vi "Test Coffee Shop Cashier Registers With Waiting to Order When Added.vi"(8 "error in (no error)":errorcluster, 11 "Coffee Shop Test in":refnum<class "Coffee Shop Test.lvclass">) -> (0 "error out":errorcluster, 3 "Coffee Shop Test out":refnum<class "Coffee Shop Test.lvclass">)   [LabVIEW 2020, in "Coffee Shop Test.lvclass"]
uses:
  Coffee Shop Test.lvclass
  C:/Program Files (x86)/National Instruments/LabVIEW 2020/vi.lib/Astemes/LUnit/Test Case.lvclass
  Processes/Coffee Shop/Coffee Shop.lvclass
  C:/Program Files (x86)/National Instruments/LabVIEW 2020/vi.lib/Astemes/Triarc Framework/Process/Process.lvclass
  Test Doubles/Mock Job Handler/Mock Job Handler.lvclass
  C:/Git/astemes-triarc-examples/Coffee Shop/Processes/People/Process Job/Job Handler.lvclass
  Processes/People/Person/Person.lvclass
  <vilib>/Astemes/Triarc Framework/Process/Process.lvclass/Process.ctl
  <vilib>/Astemes/LUnit/Test Case.lvclass/Test Case.ctl
  5b6f61c0-8826-472e-96ca-d4b217d1aee1.vi
  <vilib>/Astemes/Triarc Framework/Process/Private/SubVIs/Wait for finish.vi
  <vilib>/Astemes/Triarc Framework/Process/Private/SubVIs/Set Lifecycle State.vi
  <vilib>/Astemes/Triarc Framework/Process/Protected/Messaging/Send Message.vi
  <vilib>/Astemes/Triarc Framework/Process/Public/Lifecycle/Get Lifecycle State.vi
  <vilib>/Astemes/LUnit/Palette/Pass.vi
  <vilib>/Astemes/LUnit/Palette/Fail.vi
  <vilib>/Astemes/LUnit/Compare Variants.vi
  <vilib>/Astemes/LUnit/Describe Comparison.vi
  <vilib>/Astemes/LUnit/Set Assertion Type.vi
  <vilib>/Astemes/Triarc Framework/Process/Private/SubVIs/Handle Debug Data.vi
  <vilib>/Utility/error.llb/Clear Errors.vi
  <vilib>/Astemes/LUnit/Add test result.vi
  <vilib>/Astemes/LUnit/Variant to string.vi
  <vilib>/Astemes/Triarc Framework/Logging/Log Debug.vi
  <vilib>/AdvancedString/1D String Array to Delimited String.vi
  <vilib>/Utility/High Resolution Relative Seconds.vi
  <vilib>/Astemes/LUnit/LUnit Record Assertion Result.vi
  <vilib>/Astemes/LUnit/LUnit Aggregate Assertion Results.vi
  <vilib>/Astemes/LUnit/Method Result/LUnit Merge Status.vi
  <vilib>/Astemes/LUnit/LUnit Concatenate result strings.vi
  <vilib>/Utility/error.llb/Error Cluster From Error Code.vi
  <vilib>/Utility/Data Type/Get Type Information.vi
  <vilib>/Utility/LVClass/Get LV Class Name.vi
  <vilib>/Astemes/Triarc Framework/Process/Process.lvclass
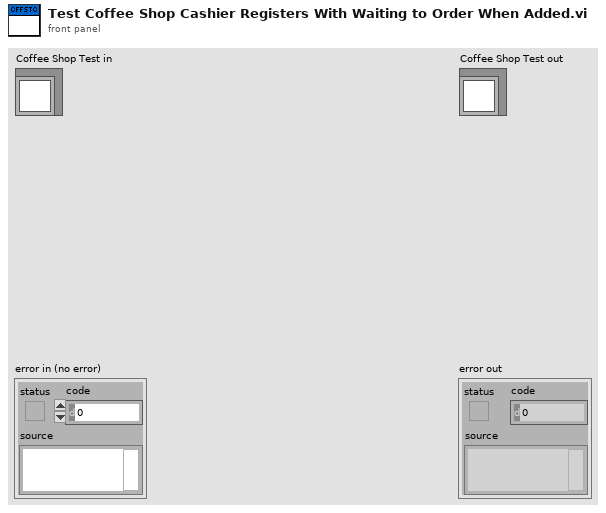
[diagram p1: front panel]
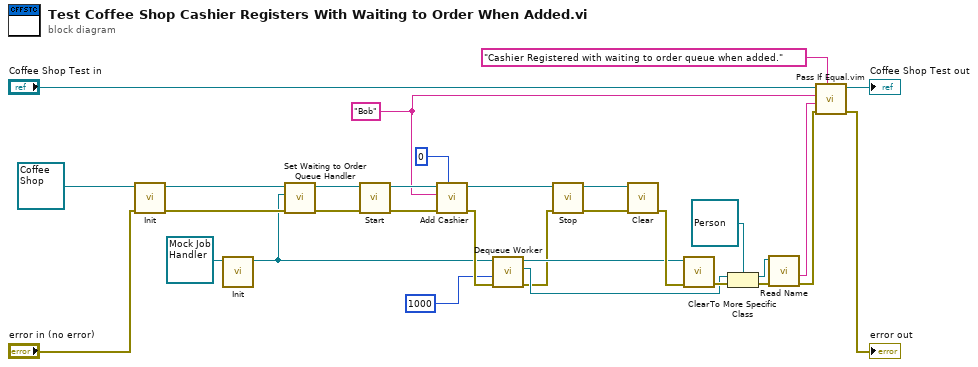
[diagram p0: block diagram]
diagram:
  w3 = "Bob" ("Name")
  n1 = call-dynamic "Init.vi"("error in (no error)"="error in (no error)", "Process In"=refnum<class "Coffee Shop.lvclass"> refnum ("Coffee Shop.lvclass")) -> ("error out"=w30:errorcluster, "Process Out"=w23:refnum<class "Coffee Shop.lvclass">)  [unwired: 8 in]
  n2 = call-dynamic "Init.vi"("Mock Job Handler In"=refnum<class "Mock Job Handler.lvclass"> refnum) -> ("Mock Job Handler Out"=w16:refnum<class "Mock Job Handler.lvclass">)  [unwired: 9 in, 1 out]
  n3 = call "Set Waiting to Order Queue Handler.vi"("error in (no error)"=w30, "Waiting To Order Queue Handler"=w16, "Coffee Shop In"=w23) -> ("error out"=w28:errorcluster, "Coffee Shop Out"=w29:refnum<class "Coffee Shop.lvclass">)  [unwired: 7 in]
  n4 = call <vilib>:"Start.vi"("error in (no error)"=w28, "Process In"=w29) -> ("error out"=w27:errorcluster, "Process Out"=w22:refnum<class "Coffee Shop.lvclass">)  [unwired: 7 in, 1 out]
  n5 = call "Add Cashier.vi"("Time Scale [ms]"=u32 0, "error in (no error)"=w27, "Name"=w3, "Coffee Shop in"=w22) -> ("error out"=w19:errorcluster, "Coffee Shop out"=w21:refnum<class "Coffee Shop.lvclass">)  [unwired: 6 in]
  n6 = call "Dequeue Worker.vi"("error in (no error)"=w19, "timeout in ms (-1)"=1000, "Mock Job Handler In"=w16) -> ("error out"=w7:errorcluster, "element"=w9:refnum<class "Job Handler.lvclass">, "Mock Job Handler Out"=w17:refnum<class "Mock Job Handler.lvclass">)  [unwired: 5 in, 1 out]
  n7 = call <vilib>:"Stop.vi"("error in (no error)"=w7, "Process In"=w21) -> ("error out"=w25:errorcluster, "Process Out"=w26:refnum<class "Coffee Shop.lvclass">)  [unwired: 7 in, 1 out]
  n8 = call-dynamic "Clear.vi"("error in (no error)"=w25, "Application In"=w26) -> ("error out"=w18:errorcluster)  [unwired: 9 in]
  n9 = call-dynamic "Clear.vi"("error in (no error)"=w18, "Mock Job Handler In"=w17) -> ("error out"=w11:errorcluster)  [unwired: 9 in]
  n10 = To More Specific Class(target class=refnum<class "Person.lvclass"> refnum ("Process In"), reference=w9) -> (specific class reference=w5:refnum<class "Person.lvclass">)  [unwired: 1 in, 1 out]
  n11 = call <vilib>:"Read Name.vi"("error in (no error)"=w11, "Process In"=w5) -> ("error out"=w6:errorcluster, "Name"=w4:string)  [unwired: 6 in, 2 out]
  n12 = call "Pass If Equal.vim"("Description"="Cashier Registered with waiting to order queue when added.", "error in (no error)"=w6, "Actual"=w4, "Expected"=w3, "LUnit Test Case In"="Coffee Shop Test in") -> ("error out"=→"error out":errorcluster, "LUnit Test Case Out"=→"Coffee Shop Test out":refnum<class "Coffee Shop Test.lvclass">)  [unwired: 5 in]
